vi "Lab11.vi"() -> ()   [LabVIEW 2022 SP3]
uses:
  <vilib>/DAQmx/write.llb/DAQmx Write (Analog DBL 1Chan 1Samp).vi
  <vilib>/DAQmx/create/channels.llb/DAQmx Create Channel (AO-Voltage-Basic).vi
  <vilib>/DAQmx/miscellaneous.llb/DAQmx Fill In Error Info.vi
panel:
  in  "stop":bool
  in  "Minimum Voltage":dbl min=-10.0 max=4.0
  in  "Maximum Voltage":dbl=10.0 min=1.0 max=10.0
  in  "Analog Voltage Out":dbl(slide) scale=0.0..5.0
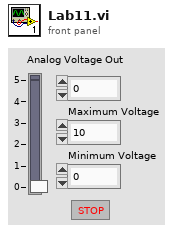
[diagram p1: front panel]
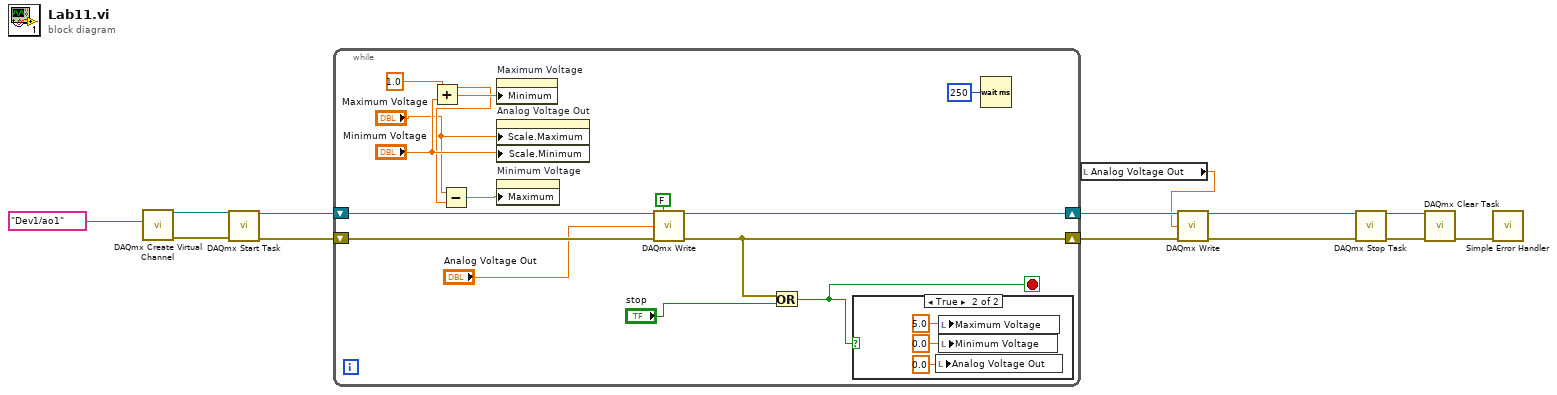
[diagram p0: block diagram]
diagram:
  n1 = call-poly <vilib>:"DAQmx Create Virtual Channel.vi"("physical channels"=tag "Dev1/ao1") -> ("task out"=w11:refnum<k21>, "error out"=w12:errorcluster)  [unwired: 13 in]
  n2 = call <vilib>:"DAQmx Start Task.vi"("task/channels in"=w11, "error in"=w12) -> ("task out"=w10:refnum<k21>, "error out"=w9:errorcluster)  [unwired: 12 in]
  n3 = while {
    shift-right: [w18] -> w5
    shift-left: w10 -> [w22]
    shift-right: [w16] -> w4
    shift-left: w9 -> [w21]
    stop <- w14 stop-if-true
    w24 = 1.0
    n4 = Add(x=w24, y="Minimum Voltage") -> (x+y=w26:dbl)
    n5 = Subtract(x="Maximum Voltage", y=w24) -> (x-y=w25:dbl)
    n6 = property on="Maximum Voltage" class="DigNum (strict)"("Minimum"=w26) -> ()  [unwired: 2 in, 2 out]
    n7 = property on="Analog Voltage Out" class="Slide (strict)"("Scale.Maximum"="Maximum Voltage", "Scale.Minimum"="Minimum Voltage") -> ()  [unwired: 2 in, 2 out]
    n8 = property on="Minimum Voltage" class="DigNum (strict)"("Maximum"=w25) -> ()  [unwired: 2 in, 2 out]
    n9 = call-poly <vilib>:"DAQmx Write.vi"("task/channels in"=w22, "auto start"=FALSE, "data"="Analog Voltage Out", "error in"=w21) -> ("task out"=w18:refnum<k21>, "error out"=w16:errorcluster)  [unwired: 9 in, 1 out]
    n10 = Or(x=w16, y="stop") -> (x .or. y?=w14:bool)
    n11 = case shown="True" w14 {
      frame False {
      }
      frame True {
        n12 = local write "Analog Voltage Out"(0.0 ("Analog Voltage Out")) -> ()
        n13 = local write "Maximum Voltage"(5.0 ("Maximum Voltage")) -> ()
        n14 = local write "Minimum Voltage"(0.0 ("Minimum Voltage")) -> ()
      }
    }
    n15 = Wait (ms)(milliseconds to wait=u32 250) -> ()  [unwired: 1 out]
  }
  n16 = local read "Analog Voltage Out"() -> (w1:dbl)
  n17 = call-poly <vilib>:"DAQmx Write.vi"("task/channels in"=w5, "data"=w1, "error in"=w4) -> ("task out"=w2:refnum<k21>, "error out"=w3:errorcluster)  [unwired: 10 in, 1 out]
  n18 = call <vilib>:"DAQmx Stop Task.vi"("task/channels in"=w2, "error in"=w3) -> ("task out"=w7:refnum<k21>, "error out"=w8:errorcluster)  [unwired: 12 in]
  n19 = call <vilib>:"DAQmx Clear Task.vi"("task in"=w7, "error in"=w8) -> ("error out"=w6:errorcluster)  [unwired: 13 in]
  n20 = call <vilib>:"Simple Error Handler.vi"("error in (no error)"=w6) -> ()  [unwired: 4 in, 5 out]
